vi "Load Telemetry.vi"(8 "error in (no error)":errorcluster, 10 "TCS telemetry":string, 11 "Acquisition in":refnum<class "Acquisition.lvclass">) -> (0 "error out":errorcluster, 3 "Acquisition out":refnum<class "Acquisition.lvclass">)   [LabVIEW 2018, in "Acquisition.lvclass"]
uses:
  Acquisition.lvclass
  Acquisition.lvclass/Acquisition.ctl
  Channel/Channel.lvclass
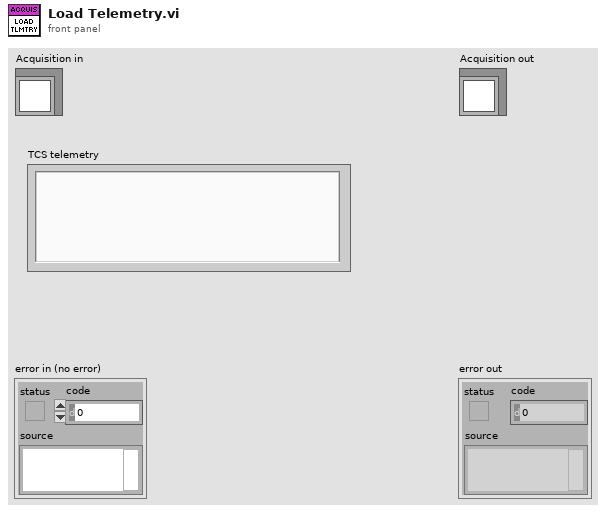
[diagram p1: front panel]
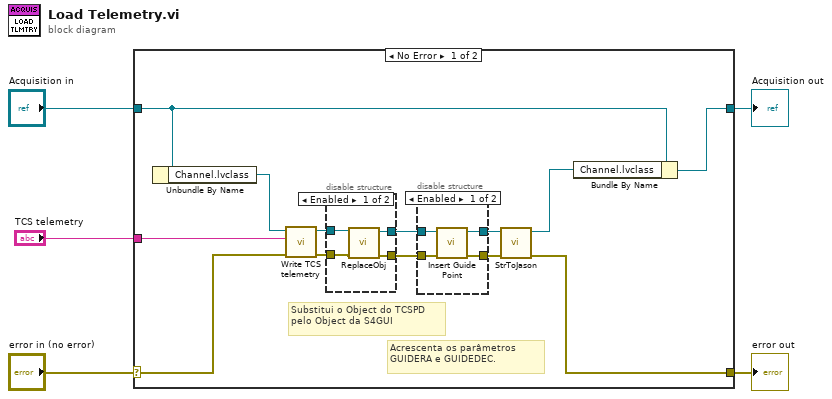
[diagram p0: block diagram]
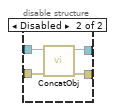
[diagram p3: hidden frame]
diagram:
  n1 = case shown="No Error" "error in (no error)" {
    selector: "error in (no error)" -> [w14 w34]
    tunnel: [w12 w34] -> w4
    tunnel: [w15 w33] -> w2
    tunnel: "Acquisition in" -> [w16 w33]
    tunnel: "TCS telemetry" -> [w18 _]
    frame No Error {
      # "Acrescenta os parâmetros GUIDERA e GUIDEDEC."
      # "Substitui o Object do TCSPD\npelo Object da S4GUI"
      n2 = Unbundle By Name(w16) -> ("Channel.lvclass"=w17:refnum<class "Channel.lvclass">)
      n3 = call-dynamic "Write TCS telemetry.vi"("error in (no error)"=w14, "TCS telemetry"=w18, "Channel in"=w17) -> ("error out"=w10:errorcluster, "Channel out"=w11:refnum<class "Channel.lvclass">)  [unwired: 7 in]
      n4 = disable-structure shown="Enabled" {
        disable-tunnel: w11 -> [w28 w32]
        disable-tunnel: [w27 w31] -> w9
        disable-tunnel: w10 -> [w26 w30]
        disable-tunnel: [w25 w29] -> w8
        frame Enabled {
          n5 = call-dynamic "ReplaceObj.vi"("error in (no error)"=w26, "Channel in"=w28) -> ("error out"=w25:errorcluster, "Channel out"=w27:refnum<class "Channel.lvclass">)  [unwired: 8 in]
        }
        frame Disabled {
          n6 = call-dynamic "ConcatObj.vi"("error in (no error)"=w30, "Channel in"=w32) -> ("error out"=w29:errorcluster, "Channel out"=w31:refnum<class "Channel.lvclass">)  [unwired: 8 in]
        }
      }
      n7 = disable-structure shown="Enabled" {
        disable-tunnel: w9 -> [w22 w24]
        disable-tunnel: w8 -> [w21 w23]
        disable-tunnel: [w20 w24] -> w7
        disable-tunnel: [w19 w23] -> w6
        frame Enabled {
          n8 = call-dynamic "Insert Guide Point.vi"("error in (no error)"=w21, "Channel in"=w22) -> ("error out"=w19:errorcluster, "Channel out"=w20:refnum<class "Channel.lvclass">)  [unwired: 8 in]
        }
        frame Disabled {
        }
      }
      n9 = call-dynamic "StrToJason.vi"("error in (no error)"=w6, "Channel in"=w7) -> ("error out"=w12:errorcluster, "Channel out"=w13:refnum<class "Channel.lvclass">)  [unwired: 7 in]
      n10 = Bundle By Name(cluster=w16, "Channel.lvclass"=w13) -> (w15:refnum<class "Acquisition.lvclass">)
    }
    frame Error {
    }
  }
  "error out" <- w4
  "Acquisition out" <- w2
